vi "is NI_DAQ Resuslt Ready.vi"(8 "error in (no error)":errorcluster, 11 "task":refnum<k21>) -> (0 "error out":errorcluster, 2 "Result Available":bool, 3 "task out":refnum<k21>)   [LabVIEW 2015]
uses:
  <resource>/objmgr/daqmx.rc
panel:
  in  "Most samples per chan":u32
  out "AvailSampPerChan":u32
  out "Done":bool
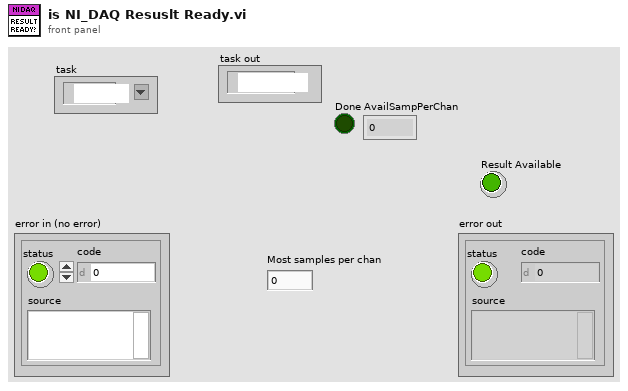
[diagram p1: front panel]
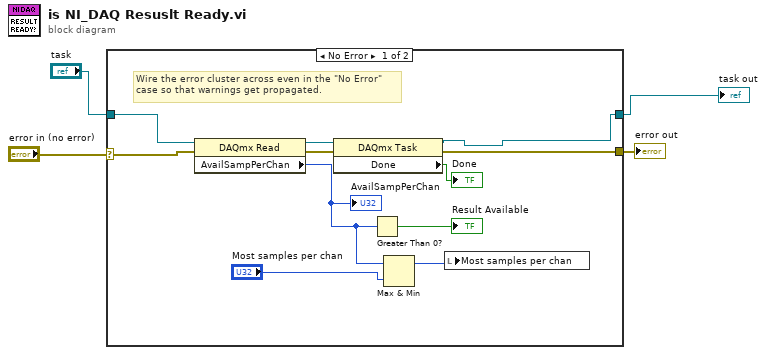
[diagram p0: block diagram]
diagram:
  n1 = case shown="No Error" "error in (no error)" {
    selector: "error in (no error)" -> [w15 w17]
    tunnel: [w12 w17] -> w3
    tunnel: [w6 w16] -> w1
    tunnel: "task" -> [w5 w16]
    frame No Error {
      # "Wire the error cluster across even in the \"No Error\"\ncase so that warnings get propagated."
      n2 = property class="DAQmx Read"(reference=w5, error in=w15) -> (reference out=w10:refnum<k21>, error out=w13:errorcluster, "AvailSampPerChan"=w9:u32)
      "AvailSampPerChan" <- w9
      n3 = property class="DAQmx Task"(reference=w10, error in=w13) -> (reference out=w6:refnum<k21>, error out=w12:errorcluster, "Done"=→"Done":bool)
      n4 = Greater Than 0?(x=w9) -> (x > 0?=→"Result Available":bool)
      n5 = Max & Min(x=w9, y="Most samples per chan") -> (max(x,y)=w7:u32)  [unwired: 1 out]
      n6 = local write "Most samples per chan"(w7) -> ()
    }
    frame Error {
    }
  }
  "error out" <- w3
  "task out" <- w1
